vi "Functional data handler.vi"(8 "error in":errorcluster, 11 "Setup cluster":T2={"Imaging Protocol"=enum."Live Imaging", "Number of Trials"=0, "Frame Size"=512, "# Averaged frames"=0, "Dwell time (us)"=0.0, "Index of Z-plane"=0, "Timelapse?"=FALSE, "Logging process is active"=FALSE, "Speed logging enabled"=FALSE, "tdms file ref"=refnum, "path"=path "", "Trial Number"=0, "Expected # points acquired"=FALSE, "Manually stopped"=FALSE, "Ch0 data"=[], "Ch1 data"=[], "Ref Data"=[], "Last trial"=FALSE, "Ref Dwell time (us)"=0.0, "# Ref Averaged frames"=0, "Ref X Length"=0, "Ref Y Length"=0, "Points acquired"={"Ch0 last trial"=0, "Ch1 last trial"=0, "All trials"=0}} {"Ref Dwell time (us)" format="%#.6g"; "Frame Size" items=["100X100"=100, "128X128"=128, "200X200"=200, "256X256"=256, "512X512"=512, "1024x1024"=1024, "2048x2048"=2048]; "Dwell time (us)" format="%#.6g"}) -> (0 "error out":errorcluster, 1 "Destination folder":path, 2 "Predominant ROI type":T1, 3 "tdms file to close":refnum<k34>)   [LabVIEW 2017]
uses:
  Typedefs/Logging queue element.ctl
  Typedefs/Imaging Protocols enum.ctl
  Typedefs/Frame Size.ctl
  Typedefs/Acquired points count.ctl
  Typedefs/ROI ID Enum.ctl
  <userlib>/_MGI/Application Control/MGI Change Detector/MGI Change Detector (T).vi
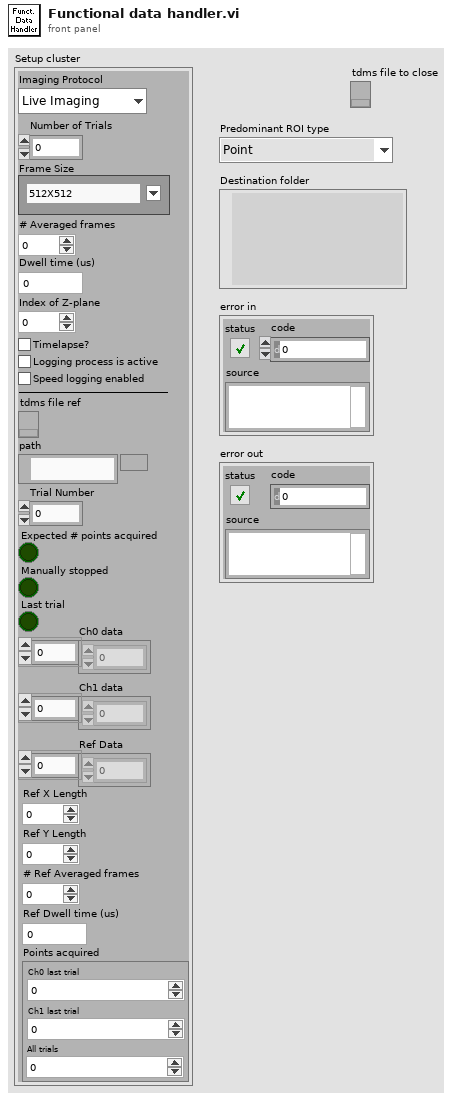
[diagram p1: front panel]
types:
  T1 = typedef "ROI ID Enum.ctl" = enum16{"Point", "MiniScan", "Comp. MiniScan", "Rectangle", "Comp. volume", "Arb. plane point"}
  T2 = typedef "Logging queue element.ctl" = cluster{"Imaging Protocol":T3, "Number of Trials":u16, "Frame Size":T4, "# Averaged frames":u16, "Dwell time (us)":dbl, "Index of Z-plane":i32, "Timelapse?":bool, "Logging process is active":bool, "Speed logging enabled":bool, "tdms file ref":refnum<k34>, "path":path, "Trial Number":i32, "Expected # points acquired":bool, "Manually stopped":bool, "Ch0 data":u32[], "Ch1 data":u32[], "Ref Data":u32[], "Last trial":bool, "Ref Dwell time (us)":dbl, "# Ref Averaged frames":u16, "Ref X Length":u16, "Ref Y Length":u16, "Points acquired":T5}
  T3 = typedef "Imaging Protocols enum.ctl" = enum16{"AOL Z-Stack", "Motor Z Stack", "Functional Acquisition", "Single Plane Acquisition", "Volume Acquisition", "Live Imaging", "Live Plane Imaging", "Live Volume Imaging"}
  T4 = typedef "Frame Size.ctl" = u16
  T5 = typedef "Acquired points count.ctl" = cluster{"Ch0 last trial":u64, "Ch1 last trial":u64, "All trials":u64}
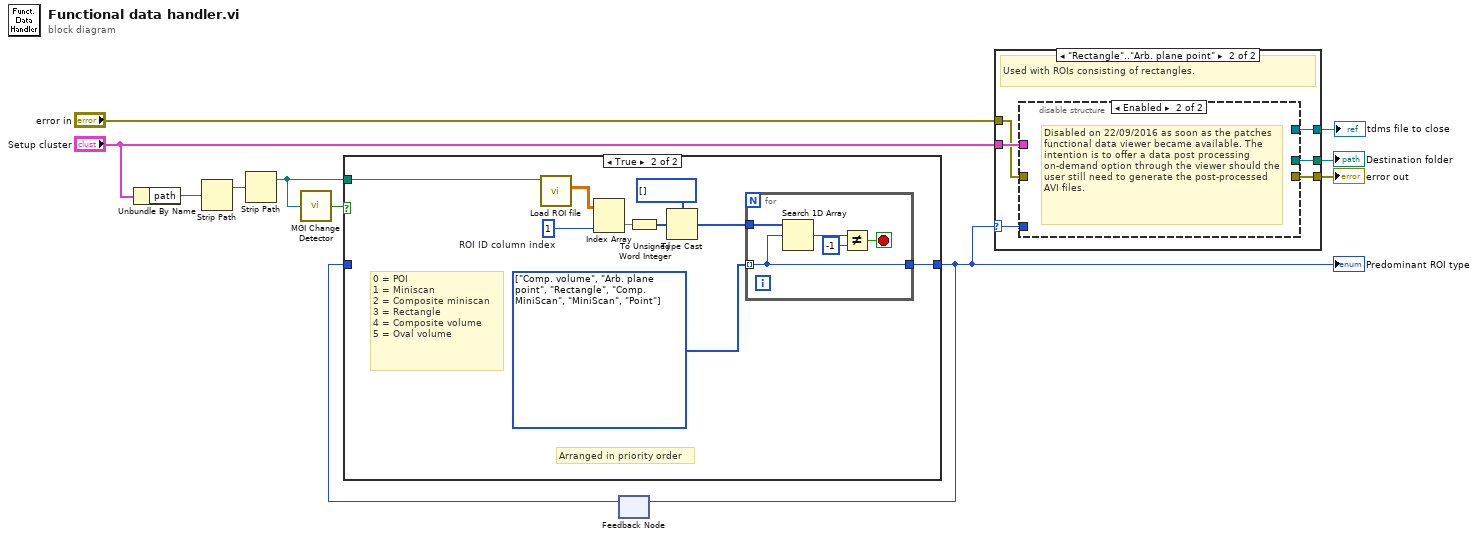
[diagram p0: block diagram]
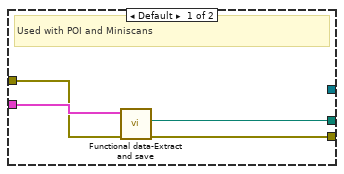
[diagram p3: hidden frame]
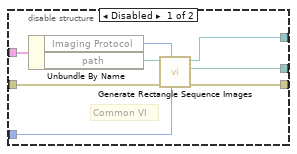
[diagram p4: hidden frame]
diagram:
  n1 = Unbundle By Name("Setup cluster") -> ("path"=w9:path)
  n2 = Strip Path(path=w9) -> (stripped path=w8:path)  [unwired: 1 out]
  n3 = Strip Path(path=w8) -> (stripped path=w4:path)  [unwired: 1 out]
  n4 = call-poly <userlib>:"MGI Change Detector.vi"("Value"=w4) -> ("Changed?"=w3:bool)
  n5 = feedback #1() -> (w1:T1)  [unwired: 1 in]
  n6 = case shown="True" w3 {
    tunnel: [w12 w20] -> w2
    tunnel: w4 -> [_ w19]
    tunnel: w1 -> [w12 _]
    frame False {
    }
    frame True {
      w15 = T1[] [] items=["Point", "MiniScan", "Comp. MiniScan", "Rectangle", "Comp. volume", "Arb. plane point"]
      w16 = 1  # ROI ID column index
      w21 = T1[] [enum."Comp. volume", enum."Arb. plane point", enum."Rectangle", enum."Comp. MiniScan", enum."MiniScan", enum."Point"] items=["Point", "MiniScan", "Comp. MiniScan", "Rectangle", "Comp. volume", "Arb. plane point"] ("*(type *) &x")
      # "Arranged in priority order"
      # "0 = POI\t \n1 = Miniscan\n2 = Composite miniscan\n3 = Rectangle\n4 = Composite volume\n5 = Oval volume"
      n7 = call "Load ROI file.vi"("Experiment data folder path"=w19) -> ("ROI Data (header removed)"=w17:dbl[][])  [unwired: 7 in, 3 out]
      n8 = Index Array(array=w17, index (col)=w16) -> (element=w13:dbl[])  [unwired: 1 in]
      n9 = To Unsigned Word Integer(number=w13) -> (unsigned 16bit integer=w14:u16[])
      n10 = Type Cast(type=w15, x=w14) -> (*(type *) &x=w18:T1[])
      n11 = for {
        tunnel: w18 -> [w26]
        tunnel: w21 -> [w22] mode=indexing
        tunnel: [w22] -> w20
        stop <- w23 stop-if-true
        n12 = Search 1D Array(1D array=w26, element=w22) -> (index of element=w25:i32)  [unwired: 1 in]
        n13 = Not Equal?(x=w25, y=-1) -> (x != y?=w23:bool)
      }
    }
  }
  "Predominant ROI type" <- w2
  n14 = feedback-in #1(w2) -> ()
  n15 = case shown="\"Rectangle\"..\"Arb. plane point\"" w2 {
    selector: w2 -> [_ w32]
    tunnel: "Setup cluster" -> [w30 w36]
    tunnel: [w29 w35] -> w11
    tunnel: [w28 w34] -> w7
    tunnel: "error in" -> [w27 w33]
    tunnel: [_ w31] -> w5
    frame Default {
      # "Used with POI and Miniscans"
      n16 = call "Functional data-Extract and save.vi"("error in (no error)"=w27, "Element received in the queue"=w30) -> ("error out"=w29:errorcluster, "Destination folder"=w28:path)  [unwired: 8 in]
    }
    frame "Rectangle".."Arb. plane point" {
      # "Used with ROIs consisting of rectangles."
      n17 = disable-structure shown="Enabled" {
        disable-tunnel: w36 -> [w44 _]
        disable-tunnel: [w42 _] -> w35
        disable-tunnel: [w41 _] -> w34
        disable-tunnel: w33 -> [w40 _]
        disable-tunnel: w32 -> [w38 _]
        disable-tunnel: [w37 _] -> w31
        frame Disabled {
          # "Common VI"
          n18 = Unbundle By Name(w44) -> ("Imaging Protocol"=w39:T3, "path"=w43:path)
          n19 = call "Generate Rectangle Sequence Images.vi"("Predominant ROI type"=w38, "Imaging Protocol"=w39, "error in (no error)"=w40, "TDMS file path & name"=w43) -> ("error out"=w42:errorcluster, "Destination fiolder"=w41:path, "tdms file to close"=w37:refnum<k34>)  [unwired: 5 in]
        }
        frame Enabled {
          # "Disabled on 22/09/2016 as soon as the patches functional data viewer became available. The intention is to offer a data post processing on-demand option through the viewer should the user still need to generate the post-processed AVI files."
        }
      }
    }
  }
  "error out" <- w11
  "Destination folder" <- w7
  "tdms file to close" <- w5
